vi "Controller Test Bench (15).vi"() -> ()   [LabVIEW 2022 SP3]
uses:
  WhiteNoise.ctl
  <vilib>/sound2/lvsound2.llb/Sound Data Format.ctl
  <vilib>/Utility/error.llb/DialogType.ctl
  <vilib>/sound2/lvsound2.llb/Sampling Mode.ctl
  <vilib>/Platform/TimedLoop/XDataNode/timing_clust.ctl
  <vilib>/Platform/TimedLoop/XDataNode/nitl_modes.ctl
  <vilib>/Platform/TimedLoop/XDataNode/wakeup.ctl
  <vilib>/sound2/lvsound2.llb/Sound File Refnum.ctl
  <vilib>/Analysis/4window.llb/windowTd.ctl
  <vilib>/DAQmx/write.llb/DAQmx Write (Analog 1D Wfm NChan NSamp).vi
  <vilib>/DAQmx/read.llb/DAQmx Read (Analog 1D Wfm NChan NSamp).vi
  <vilib>/DAQmx/create/channels.llb/DAQmx Create Channel (AI-Acceleration-Accelerometer).vi
  <vilib>/DAQmx/configure/timing.llb/DAQmx Timing (Sample Clock).vi
  <vilib>/Platform/TimedLoop/scheduler/LVUserAPI/_suppVIs/Create_1kHz_TSource.vi
  <vilib>/DAQmx/create/channels.llb/DAQmx Create Channel (AO-Voltage-Basic).vi
  <vilib>/sound2/lvsound2.llb/Sound File Info (path).vi
  <vilib>/sound2/lvsound2.llb/Sound File Read Open.vi
  <vilib>/sound2/lvsound2.llb/Sound Output Set Volume (Single).vi
  <vilib>/sound2/lvsound2.llb/Sound File Read (DBL).vi
  <vilib>/sound2/lvsound2.llb/Sound Output Write (DBL).vi
  <vilib>/DAQmx/miscellaneous.llb/DAQmx Fill In Error Info.vi
  <vilib>/DAQmx/configure/task.llb/DAQmx Configure Logging (TDMS).vi
  <vilib>/measure/maspectr.llb/FFT Spectrum (Mag-Phase) for N Chan.vi
  <vilib>/platform/TimedLoop/XDataNode/XDataNode.xnode
  <vilib>/measure/NI_MAPro.lvlib
  <resource>/objmgr/daqmx.rc
  <vilib>/Analysis/NI_AALPro.lvlib
  <vilib>/measure/NI_MABase.lvlib
  <vilib>/addons/control/pid/NI_PID_pid.lvlib
  <vilib>/Platform/TimedLoop/XDataNode/XDNodeRunTimeDep.lvlib
  <vilib>/addons/control/pid/pid.llb/PID (DBL Array).vi
panel:
  in  "Time Out (s)":dbl=1000.0
  out "Elapsed Time":i32 caption="Elapsed Time (s)" format="%.2f"
  in  "Time Out (s)":dbl=1000.0
  out "Active Controller Output":dbl[](graph)
  out "Elapsed Time":i32 caption="Elapsed Time (s)" format="%.2f"
  in  "Acquisition\nPeriod(ms)":dbl=41.2
  out "Accel.1":waveform(dbl)[](graph)
  out "Excitation Output":waveform(dbl)[](graph)
  in  "Output Noise":bool=TRUE
  in  "?":T1(tab)=enum."Harmonic"
  in  "Cluster 3":T2={"Path txt/csv File"=path "C:/Users/LAV-UFSC-2023/Documents/LAV-TCC/Dados-Experimentos/acc_time/Previous Data/handlebar_acc1_run2.txt", "Delimiter"=".", "Separator"="\\t", "Offset (lines)"=21.0}
  in  "Gain":i32
  in  "Stop 3":bool
  in  "Gain":i32
  in  "Cluster 4":T4={"Seed"=0.0, "Iterator"=1.0, "Path Sound File"=path "C:/Users/LAV-UFSC-2023/Documents/LAV-TCC/Dados-Experimentos/Dados Empíricos/Uni-cheio.wav", "number of samples/ch (-1: all)"=-1}
  in  "Stop 2":bool
  in  "Cluster":T5={"Seed"=0.0, "Standard Deviation"=0.2, "Reset"=FALSE, "Iterator"=1.0, "Seed"=-1, "Stop 4"=FALSE, "Lower Cut-Off 2"=5.0, "Upper Cut-Off 2"=350.0} {"Upper Cut-Off 2" min=5.0 max=350.0 step=10.0; "Lower Cut-Off 2" min=5.0 max=350.0 step=10.0; "Standard Deviation" min=0.001 max=1.5 step=0.05 format="%0.2p"}
  in  "Cluster 2":T6={"Iterator"=1.0, "Waveform Type"=0, "Frequency"=10.0, "Amplitude"=0.25, "Stop 4"=FALSE} {"Frequency" min=5.0 max=350.0 step=10.0 format="%0.2p"; "Waveform Type" items=["Sine Wave", "Triangle Wave", "Square Wave", "Sawtooth Wave"]; "Amplitude" min=0.001 max=0.3 step=0.05 format="%0.2p"}
  in  "Active Control":bool
  in  "Tab Control":T7(tab)
  out "dt out (s)":dbl format="%.3f"
  in  "setpoint":dbl[](array[numeric])=[0.0] format="%.2f"
  in  "PID gains":T8(array[cluster])=[{"proportional gain (Kc)"=1.0, "integral time (Ti, min)"=0.01, "derivative time (Td, min)"=0.0}] {"derivative time (Td, min)" format="%.3e"; "integral time (Ti, min)" format="%.3e"; "proportional gain (Kc)" step=0.0025 format="%.3e"}
  in  "dt (s)":dbl=-1.0 format="%.3f"
  in  "output range":cluster{"output high":dbl, "output low":dbl}[](array[cluster])=[{"output high"=100.0, "output low"=-100.0}] {"output low" format="%.2f"; "output high" format="%.2f"}
  in  "Upper Cut-Off":dbl=400.0
  in  "Lower Cut-Off":dbl=100.0
  in  "Setpoint":dbl
  in  "Gain":dbl min=0.0 step=0.01
  out "Output Signal":dynamicdata(graph)
  in  "Upper Cut-Off":dbl=400.0
  in  "Lower Cut-Off":dbl=100.0
  out "Accel.2":waveform(dbl)[](graph)
  in  "Log Raw Data":bool
  out "Mag 2":cluster{"f0":dbl, "df":dbl, "magnitude":dbl[]}[](graph)
  in  "Show FFT":bool=TRUE
  in  "Log FFT":bool
  in  "Start Reading":bool=TRUE
  in  "Stop":bool
  # "Active Controller"
  # "Main\nSwitch"
  # "Output Noise"
  # "RAW - Accel. 1"
  # "Data Acquisition"
  # "FFT - Amplitude (dB)"
  # "RAW - Accel. 2"
  # "Runtime"
  # "Pre-Set"
  # "Runtime"
  # "Pre-Set"
  # "Runtime"
  # "Filter"
  # "Runtime"
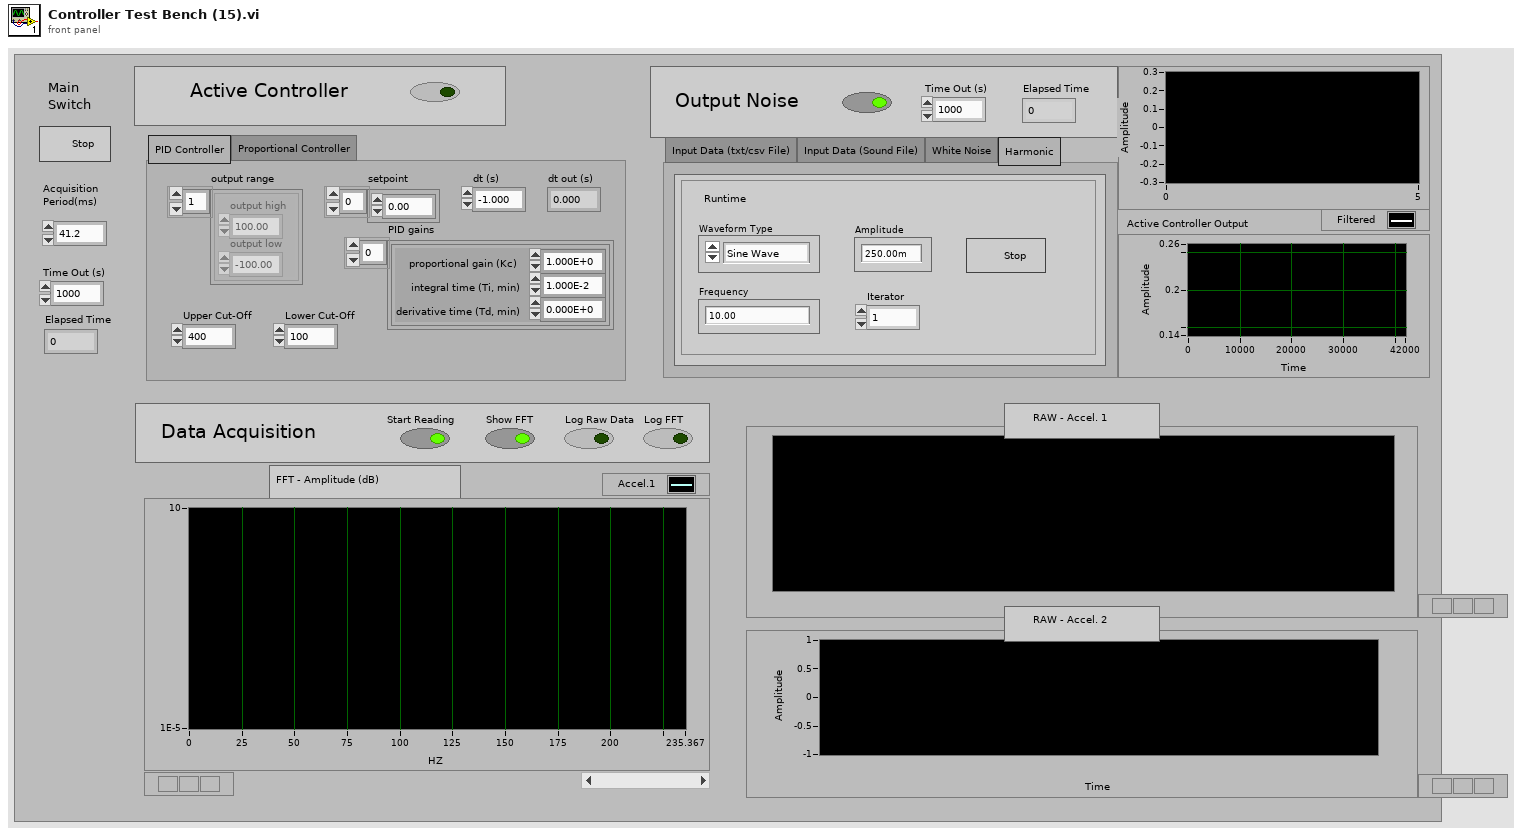
[diagram p1: front panel]
types:
  T1 = enum32{"Input Data (txt/csv File)", "Input Data (Sound File)", "White Noise", "Harmonic"}
  T2 = cluster{"Path txt/csv File":path, "Delimiter":string, "Separator":string, "Offset (lines)":dbl}
  T3 = typedef "WhiteNoise.ctl" = dbl
  T4 = cluster{"Seed":T3, "Iterator":dbl, "Path Sound File":path, "number of samples/ch (-1: all)":i32}
  T5 = cluster{"Seed":T3, "Standard Deviation":dbl, "Reset":bool, "Iterator":dbl, "Seed":i8, "Stop 4":bool, "Lower Cut-Off 2":dbl, "Upper Cut-Off 2":dbl}
  T6 = cluster{"Iterator":dbl, "Waveform Type":u16, "Frequency":dbl, "Amplitude":dbl, "Stop 4":bool}
  T7 = enum32{"PID Controller", "Proportional Controller"}
  T8 = cluster{"proportional gain (Kc)":dbl, "integral time (Ti, min)":dbl, "derivative time (Td, min)":dbl}[]
  T9 = typedef "Sampling Mode.ctl" = i32
  T10 = typedef "DialogType.ctl" = u16
  T11 = typedef "Sound Data Format.ctl" = cluster{"sample rate (S/s)":dbl, "number of channels":i32, "bits per sample":i32}
  T12 = typedef "Sound Output Task ID.ctl" = u32
  T13 = typedef "XDNodeRunTimeDep.lvlib/timing_clust.ctl" = cluster{"Expected End [f-1]":u64, "Actual End [f-1]":u64, "Finished Late? [f-1]":bool, "Expected End [i-1]":u64, "Actual End [i-1]":u64, "Finished Late? [i-1]":bool, "Expected Start [i]":u64, "Actual Start [i]":u64, "Expected Start [f]":u64, "Actual Start [f]":u64, "Source Name":string, "Structure Name":string, "Period":i64, "Deadline":i64, "Offset":i64, "Start":i64, "Priority":i32, "Timeout":i32, "Mode":T14, "Wakeup Reason":T15, "Error":errorcluster, "Source Type":string, "Secondary Source Type":string, "Global End Time":u64, "Global Start Time":u64, "Frame Duration":u64, "Iteration Duration":u64, "Assigned CPU":i32, "I/O Scan Engine Mode":u32}
  T14 = typedef "XDNodeRunTimeDep.lvlib/nitl_modes.ctl" = enum32{"No Change", "Process missed periods, maintain original phase", "Discard missed periods, maintain original phase", "Process missed periods, ignore original phase", "Discard missed periods, ignore original phase"}
  T15 = typedef "XDNodeRunTimeDep.lvlib/wakeup.ctl" = enum32{"Normal", "Aborted", "Asynchronous wakeup", "Timing source error", "Timed loop error", "Timeout"}
  T16 = typedef "Sound File Refnum.ctl" = refnum<file>
  T17 = typedef "NI_AALPro.lvlib/windowTd.ctl" = u32
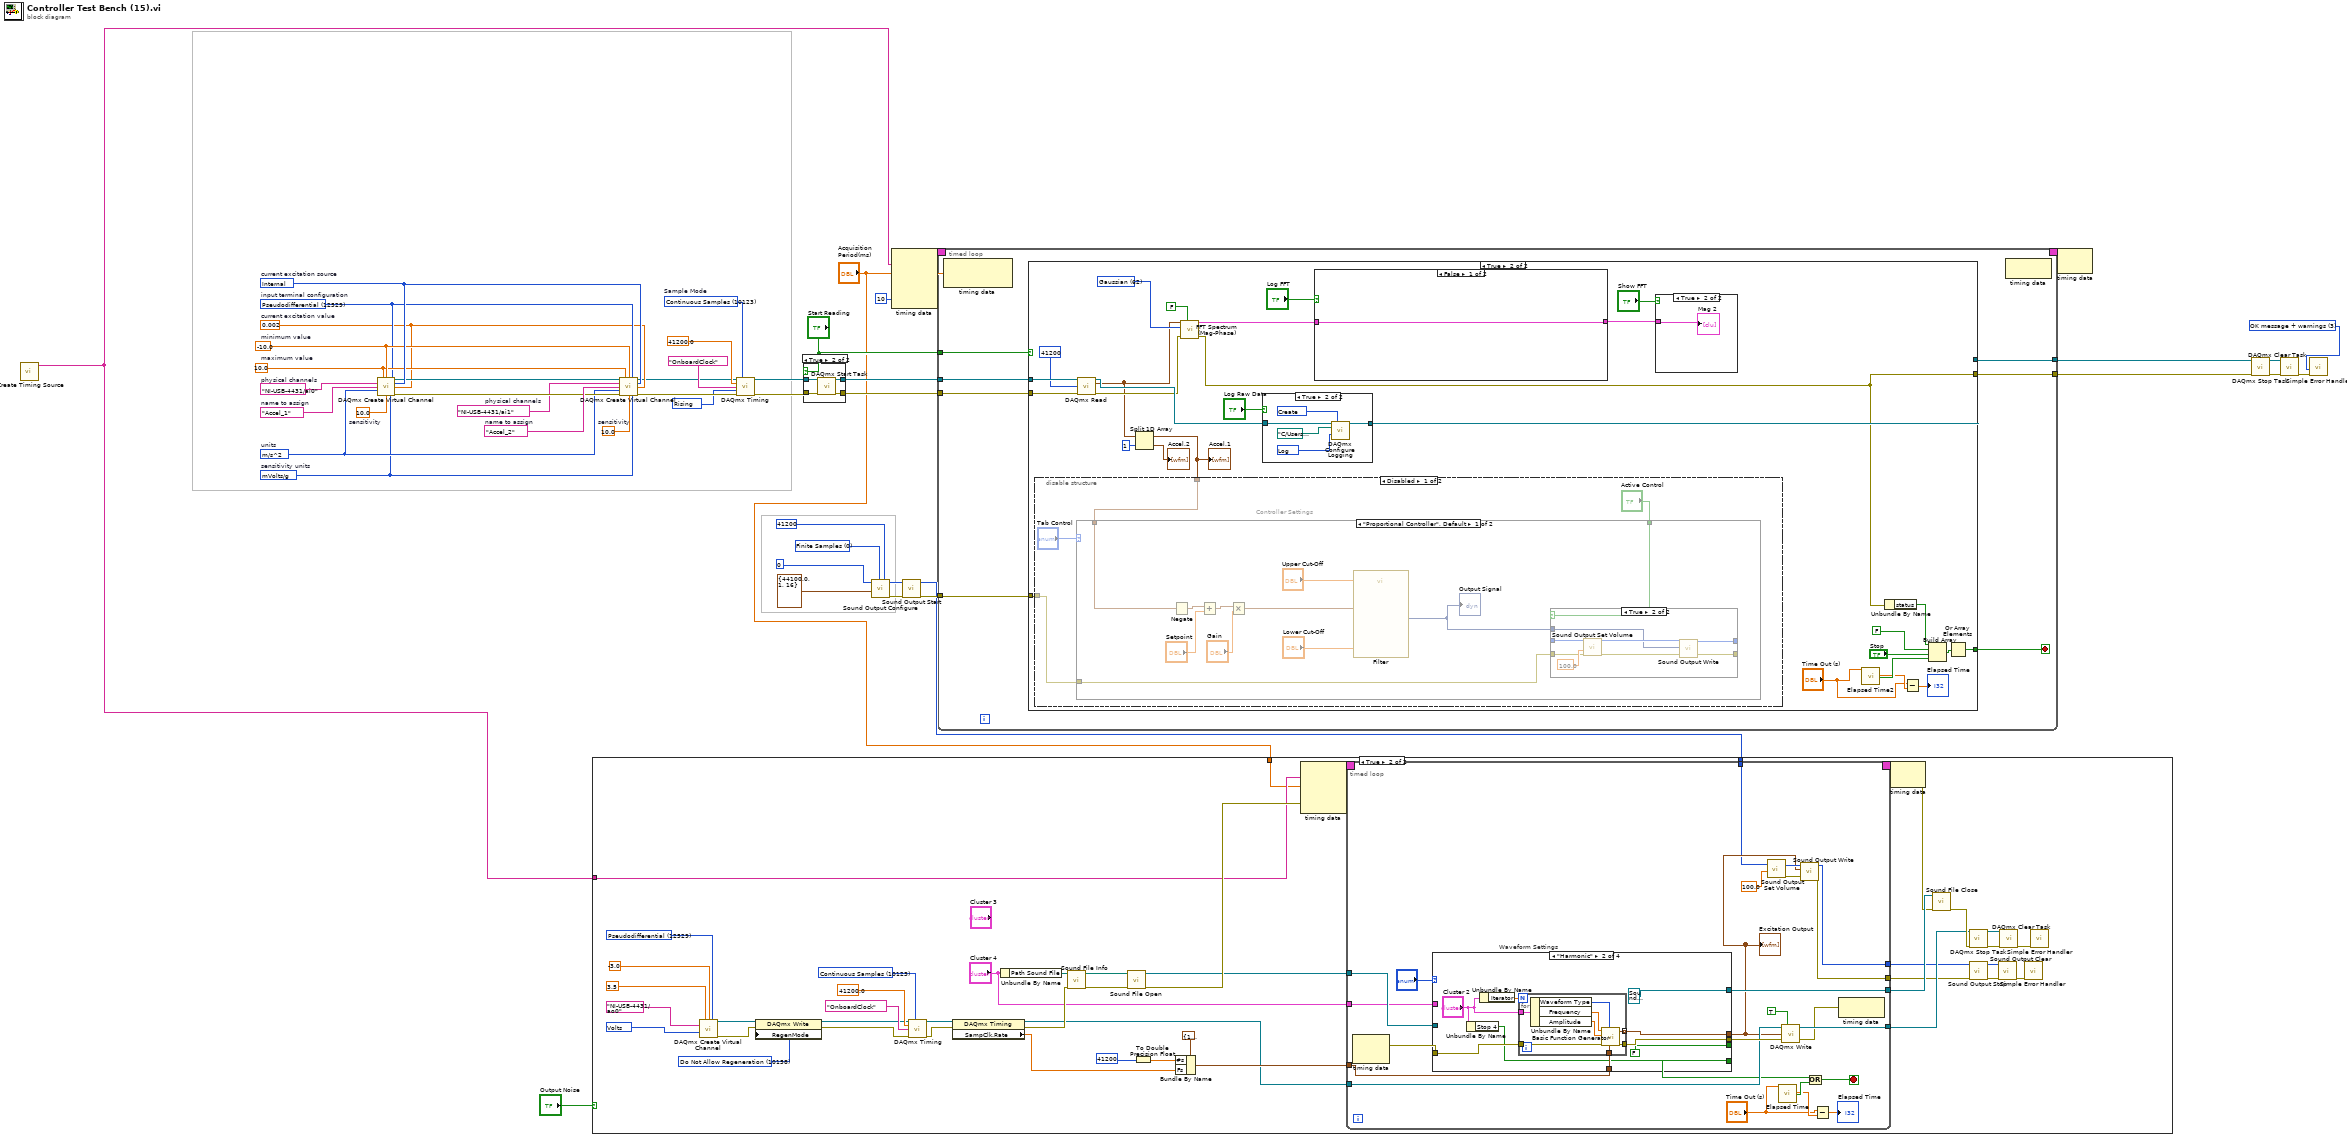
[diagram p0: block diagram]
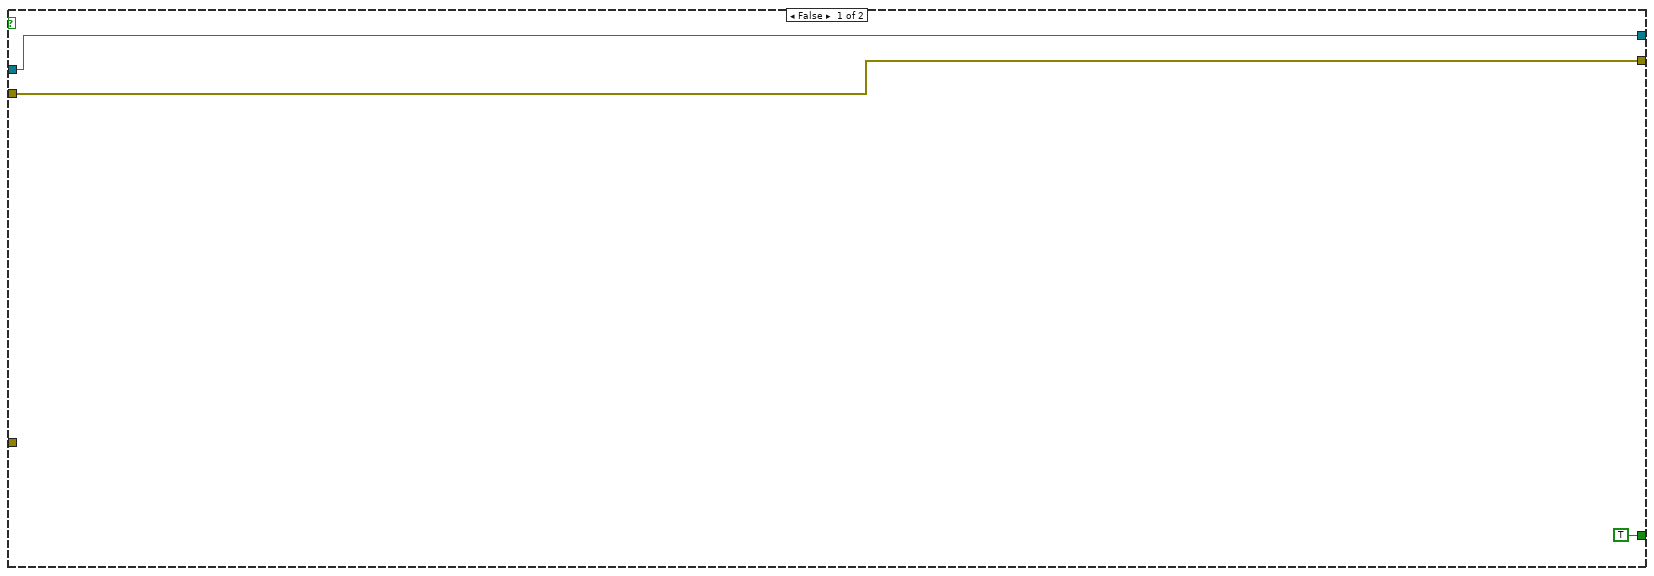
[diagram p2: hidden frame]
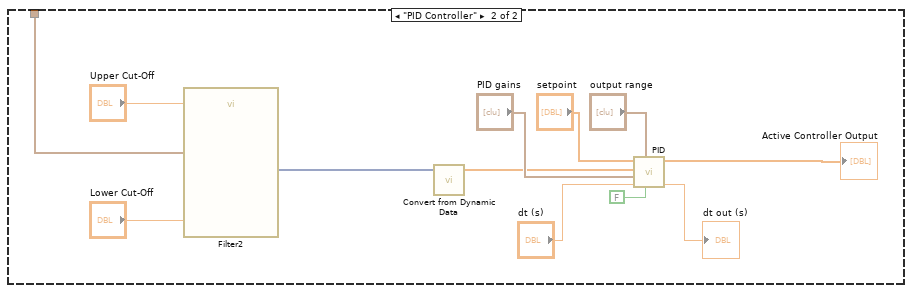
[diagram p4: hidden frame]
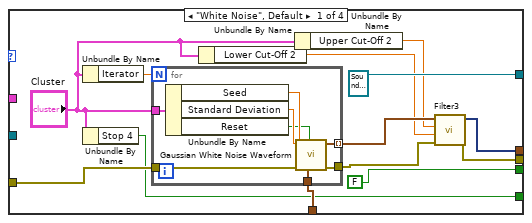
[diagram p10: hidden frame]
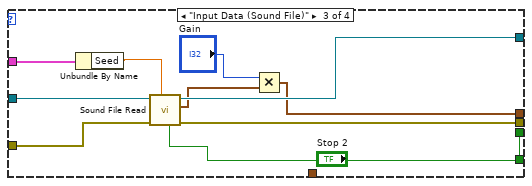
[diagram p11: hidden frame]
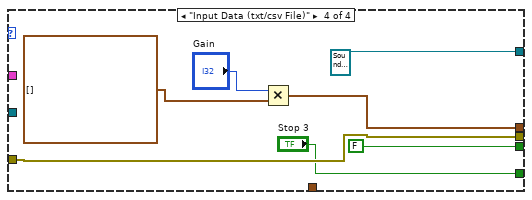
[diagram p12: hidden frame]
diagram:
  w4 = 10280 items=["Rising"=10280, "Falling"=10171] ("active edge")
  w6 = 12509 items=["mVolts/g"=12509, "Volts/g"=12510]  # sensitivity units
  w35 = 10.0  # sensitivity
  w5 = 0.002  # current excitation value
  w29 = 10200 items=["Internal"=10200, "External"=10167, "None"=10230]  # current excitation source
  w21 = tag "NI-USB-4431/ai0"  # physical channels
  w34 = 10123 items=["Finite Samples"=10178, "Continuous Samples"=10123, "Hardware Timed Single Point"=12522]  # Sample Mode
  w24 = 12529 items=["default"=-1, "RSE"=10083, "NRSE"=10078, "Differential"=10106, "Pseudodifferential"=12529]  # input terminal configuration
  w27 = -10.0  # minimum value
  w26 = 10.0  # maximum value
  w36 = "Accel_1"  # name to assign
  w25 = 12470 items=["g"=10186, "m/s^2"=12470, "in/s^2"=12471, "From Custom Scale"=10065]  # units
  w37 = 10.0  # sensitivity
  w22 = tag "NI-USB-4431/ai1"  # physical channels
  w31 = "Accel_2"  # name to assign
  w38 = T9 0 items=["Finite Samples", "Continuous Samples"] ("sample mode")
  w39 = T10 3 items=["no dialog", "OK message", "continue or stop message", "OK message + warnings", "continue/stop + warnings"] ("type of dialog (OK msg:1)")
  n1 = call-poly <vilib>:"Create Timing Source.vi"() -> ("name (out)"=w13:string)  [unwired: 10 in, 1 out]
  n2 = call-poly <vilib>:"DAQmx Create Virtual Channel.vi"("maximum value"=w26, "minimum value"=w27, "input terminal configuration"=w24, "physical channels"=w21, "current excitation source"=w29, "name to assign"=w36, "current excitation value"=w5, "units"=w25, "sensitivity"=w35, "sensitivity units"=w6) -> ("task out"=w23:refnum<k21>, "error out"=w30:errorcluster)  [unwired: 4 in]
  n3 = call-poly <vilib>:"DAQmx Create Virtual Channel.vi"("task in"=w23, "maximum value"=w26, "minimum value"=w27, "input terminal configuration"=w24, "physical channels"=w22, "current excitation source"=w29, "name to assign"=w31, "current excitation value"=w5, "units"=w25, "error in"=w30, "sensitivity"=w37, "sensitivity units"=w6) -> ("task out"=w2:refnum<k21>, "error out"=w28:errorcluster)  [unwired: 2 in]
  n4 = call-poly <vilib>:"DAQmx Timing.vi"("task/channels in"=w2, "sample mode"=w34, "rate"=41200.0 ("Sample Rate"), "source"=tag "OnboardClock" ("Sample Clock Source"), "active edge"=w4, "error in"=w28) -> ("task out"=w19:refnum<k21>, "error out"=w20:errorcluster)  [unwired: 8 in]
  n5 = case shown="True" "Start Reading" {
    tunnel: w20 -> [w47 w52]
    tunnel: w19 -> [w48 w51]
    tunnel: [w48 w50] -> w10
    tunnel: [w47 w49] -> w11
    frame False {
    }
    frame True {
      n6 = call <vilib>:"DAQmx Start Task.vi"("task/channels in"=w51, "error in"=w52) -> ("task out"=w50:refnum<k21>, "error out"=w49:errorcluster)  [unwired: 12 in]
    }
  }
  n7 = call <vilib>:"Sound Output Configure.vi"("number of samples/ch"=41200 ("Number of Samples/ch"), "sample mode"=w38, "sound format"=T11 {"sample rate (S/s)"=44100.0, "number of channels"=1, "bits per sample"=16} ("Sound Format"), "device ID"=u32 0 ("Device ID")) -> ("error out"=w18:errorcluster, "task ID"=w17:T12)  [unwired: 6 in]
  n8 = node-c288(w13, "Acquisition\nPeriod(ms)", i64 10 ("Offset")) -> (w15:T13)  [unwired: 2 in]
  n9 = call <vilib>:"Sound Output Start.vi"("error in (no error)"=w18, "task ID"=w17) -> ("error out"=w12:errorcluster, "task ID out"=w1:T12)  [unwired: 8 in]
  n10 = case shown="True" "Output Noise" {
    tunnel: w13 -> [_ w69]
    tunnel: "Acquisition\nPeriod(ms)" -> [_ w59]
    tunnel: w1 -> [_ w53]
    frame False {
    }
    frame True {
      w85 = 10123 items=["Finite Samples"=10178, "Continuous Samples"=10123, "Hardware Timed Single Point"=12522] ("sample mode")
      w89 = 10158 items=["Allow Regeneration"=10097, "Do Not Allow Regeneration"=10158] ("RegenMode")
      w95 = 12529 items=["Default"=-1, "RSE"=10083, "Differential"=10106, "Pseudodifferential"=12529] ("output terminal configuration")
      w93 = 10348 items=["Volts"=10348, "From Custom Scale"=10065] ("units")
      n11 = call-poly <vilib>:"DAQmx Create Virtual Channel.vi"("maximum value"=3.5, "minimum value"=-3.0, "output terminal configuration"=w95, "physical channels"=tag "NI-USB-4431/ao0", "units"=w93) -> ("task out"=w88:refnum<k21>, "error out"=w90:errorcluster)  [unwired: 9 in]
      n12 = property class="DAQmx Write"(reference=w88, error in=w90, "RegenMode"=w89) -> (reference out=w86:refnum<k21>, error out=w87:errorcluster)
      n13 = call-poly <vilib>:"DAQmx Timing.vi"("task/channels in"=w86, "sample mode"=w85, "rate"=41200.0 ("Sample Rate"), "source"=tag "OnboardClock" ("Sample Clock Source"), "error in"=w87) -> ("task out"=w81:refnum<k21>, "error out"=w80:errorcluster)  [unwired: 9 in]
      n14 = property class="DAQmx Timing"(reference=w81, error in=w80) -> (reference out=w64:refnum<k21>, error out=w74:errorcluster, "SampClk.Rate"=w82:dbl)
      n15 = Unbundle By Name("Cluster 4") -> ("Path Sound File"=w62:path)
      n16 = call-poly <vilib>:"Sound File Info.vi"("error in (no error)"=w74, "path"=w62) -> ("error out"=w76:errorcluster, "path out"=w75:path)  [unwired: 6 in, 2 out]
      n17 = call-poly <vilib>:"Sound File Open.vi"("error in (no error)"=w76, "path"=w75) -> ("error out"=w70:errorcluster, "sound file refnum"=w68:T16)  [unwired: 8 in]
      n18 = To Double Precision Float(number=41200) -> (double precision float=w83:dbl)
      n19 = Bundle By Name(cluster=cluster{"Fs":dbl, "#s":dbl} {"Fs"=1000.0, "#s"=1000.0} ("sampling info"), "#s"=w83, "Fs"=w82) -> (w65:cluster{"Fs":dbl, "#s":dbl})
      n20 = node-c288(w69, w59, w70) -> (w72:T13)  [unwired: 1 in]
      n21 = timed-loop {
        timing: w72 -> [_]
        timing-out: [_] -> w71
        tunnel: w68 -> [w117]
        tunnel: [w116] -> w67
        tunnel: [w115] -> w66
        tunnel: w65 -> [w114]
        tunnel: w64 -> [w113]
        tunnel: "Cluster 4" -> [w112]
        tunnel: [w100] -> w55
        tunnel: [w99] -> w54
        tunnel: w53 -> [w98]
        stop <- w111 stop-if-true
        # "Waveform Settings"
        n22 = node-c288() -> (w118:errorcluster)  [unwired: 1 in, 1 out]
        n23 = case shown="\"Harmonic\"" "?" {
          tunnel: w114 -> [w134 w149 _ _]
          tunnel: w118 -> [w132 w151 w170 w175]
          tunnel: [w125 w148 w169 w175] -> w120
          tunnel: [w127 w150 w165 w171] -> w101
          tunnel: w117 -> [_ _ w168 _]
          tunnel: [FALSE FALSE w167 FALSE ("end of file?")] -> _
          tunnel: [T16 refnum ("sound file refnum out") T16 refnum ("sound file refnum out") w166 T16 refnum ("sound file refnum out")] -> w116
          tunnel: w112 -> [_ _ w162 _]
          tunnel: [w129 w143 "Stop 2" "Stop 3"] -> w110
          frame "White Noise", Default {
            n24 = Unbundle By Name("Cluster") -> ("Iterator"=w133:dbl)
            n25 = Unbundle By Name("Cluster") -> ("Stop 4"=w129:bool)
            n26 = for {
              N: w133 -> [_]
              tunnel: w132 -> [w142]
              tunnel: w134 -> [w141]
              tunnel: [w140] -> w126
              tunnel: "Cluster" -> [w139]
              tunnel: [w138] -> w128 mode=indexing
              n27 = Unbundle By Name(w139) -> ("Seed"=w137:T3, "Standard Deviation"=w136:dbl, "Reset"=w135:bool)
              n28 = call <vilib>:"Gaussian White Noise Waveform.vi"("sampling info"=w141, "reset signal"=w135, "error in (no error)"=w142, "seed"=w137, "standard deviation"=w136) -> ("error out"=w140:errorcluster, "signal out"=w138:waveform(dbl))  [unwired: 5 in]
            }
            n29 = Unbundle By Name("Cluster") -> ("Lower Cut-Off 2"=w123:dbl)
            n30 = Unbundle By Name("Cluster") -> ("Upper Cut-Off 2"=w122:dbl)
            n31 = call "Filter3"("error in (no error)"=w126, "Lower Cut-Off"=w123, "Upper Cut-Off"=w122, "Signal"=w128) -> ("error out"=w125:errorcluster, "Filtered Signal"=w127:dynamicdata)  [unwired: 6 in]
          }
          frame "Harmonic" {
            n32 = Unbundle By Name("Cluster 2") -> ("Stop 4"=w143:bool)
            n33 = Unbundle By Name("Cluster 2") -> ("Iterator"=w147:dbl)
            n34 = for {
              N: w147 -> [_]
              tunnel: w151 -> [w159]
              tunnel: w149 -> [w158]
              tunnel: [w157] -> w148
              tunnel: "Cluster 2" -> [w156]
              tunnel: [w152] -> w150 mode=indexing
              n35 = Unbundle By Name(w156) -> ("Waveform Type"=w155:u16, "Frequency"=w154:dbl, "Amplitude"=w153:dbl)
              n36 = call <vilib>:"Basic Function Generator.vi"("sampling info"=w158, "signal type"=w155, "error in (no error)"=w159, "amplitude"=w153, "frequency"=w154) -> ("error out"=w157:errorcluster, "signal out"=w152:waveform(dbl))  [unwired: 4 in, 1 out]
            }
          }
          frame "Input Data (Sound File)" {
            n37 = Unbundle By Name(w162) -> ("Seed"=w163:T3)
            n38 = call-poly <vilib>:"Sound File Read.vi"("number of samples/ch (-1: all)"=w163, "error in (no error)"=w170, "sound file refnum"=w168) -> ("error out"=w169:errorcluster, "data"=w164:waveform(dbl)[], "sound file refnum out"=w166:T16, "end of file?"=w167:bool)  [unwired: 4 in, 1 out]
            n39 = Multiply(x="Gain", y=w164) -> (x*y=w165:waveform(dbl)[])
          }
          frame "Input Data (txt/csv File)" {
            n40 = Multiply(x="Gain", y=waveform(dbl)[] []) -> (x*y=w171:waveform(dbl)[])
          }
        }
        "Excitation Output" <- w101
        n41 = call-poly <vilib>:"Sound Output Set Volume.vi"("volume"=100.0, "task ID"=w98) -> ("error out"=w102:errorcluster, "task ID out"=w103:T12)  [unwired: 8 in]
        n42 = call "Elapsed Time"("Time Target (s)"="Time Out (s)") -> ("Elapsed Time (s)"=w106:dbl, "Time has Elapsed"=w107:bool)  [unwired: 11 in, 6 out]
        n43 = call-poly <vilib>:"DAQmx Write.vi"("task/channels in"=w113, "auto start"=TRUE, "data"=w101, "error in"=w120) -> ("task out"=w115:refnum<k21>, "error out"=w109:errorcluster)  [unwired: 9 in, 1 out]
        n44 = call-poly <vilib>:"Sound Output Write.vi"("error in (no error)"=w102, "data"=w101, "task ID"=w103) -> ("error out"=w99:errorcluster, "task ID out"=w100:T12)  [unwired: 7 in]
        n45 = Or(x=w110, y=w107) -> (x .or. y?=w111:bool)
        n46 = Subtract(x="Time Out (s)", y=w106) -> (x-y=→"Elapsed Time":dbl)
        n47 = node-c288(w109) -> ()  [unwired: 1 out]
      }
      n48 = node-c288(w71) -> (w60:errorcluster)
      n49 = call <vilib>:"Sound File Close.vi"("error in (no error)"=w60, "sound file refnum"=w67) -> ("error out"=w73:errorcluster)  [unwired: 9 in]
      n50 = call <vilib>:"DAQmx Stop Task.vi"("task/channels in"=w66, "error in"=w73) -> ("task out"=w79:refnum<k21>, "error out"=w78:errorcluster)  [unwired: 12 in]
      n51 = call <vilib>:"Sound Output Stop.vi"("error in (no error)"=w54, "task ID"=w55) -> ("error out"=w56:errorcluster, "task ID out"=w57:T12)  [unwired: 8 in]
      n52 = call <vilib>:"Sound Output Clear.vi"("error in (no error)"=w56, "task ID"=w57) -> ("error out"=w58:errorcluster)  [unwired: 9 in]
      n53 = call <vilib>:"DAQmx Clear Task.vi"("task in"=w79, "error in"=w78) -> ("error out"=w77:errorcluster)  [unwired: 13 in]
      n54 = call <vilib>:"Simple Error Handler.vi"("error in (no error)"=w58) -> ()  [unwired: 4 in, 5 out]
      n55 = call <vilib>:"Simple Error Handler.vi"("error in (no error)"=w77) -> ()  [unwired: 4 in, 5 out]
    }
  }
  n56 = timed-loop {
    timing: w15 -> [_]
    timing-out: [_] -> w14
    tunnel: "Start Reading" -> [w196]
    tunnel: w12 -> [w195]
    tunnel: w11 -> [w194]
    tunnel: w10 -> [w193]
    tunnel: [w192] -> w9
    tunnel: [w191] -> w8
    stop <- w190 stop-if-true
    n57 = node-c288() -> ()  [unwired: 1 in, 2 out]
    n58 = case shown="True" w196 {
      tunnel: w193 -> [w199 w227]
      tunnel: w194 -> [w198 w226]
      tunnel: [w199 w223] -> w191
      tunnel: [w198 w214] -> w192
      tunnel: w195 -> [_ w208]
      tunnel: [TRUE w205] -> w190
      frame False {
      }
      frame True {
        w213 = T17 62 items=["Rectangle"=0, "Hanning"=1, "Hamming"=2, "Blackman-Harris"=3, "Exact Blackman"=4, "Blackman"=5, "Flat Top"=6, "4 Term B-Harris "=7, "7 Term B-Harris"=8, "Low Sidelobe"=9, "Blackman Nuttall"=11, "Triangle"=30, "Bartlett-Hanning"=31, "Bohman"=32, "Parzen"=33, "Welch"=34, "Kaiser"=60, "Dolph-Chebyshev"=61, "Gaussian"=62] ("window")
        n59 = call-poly <vilib>:"DAQmx Read.vi"("task/channels in"=w227, "number of samples per channel"=41200, "error in"=w226) -> ("task out"=w224:refnum<k21>, "data"=w207:waveform(dbl)[], "error out"=w215:errorcluster)  [unwired: 10 in]
        n60 = Split 1D Array(array=w207, index=1) -> (first subarray=w206:waveform(dbl)[], second subarray=→"Accel.2":waveform(dbl)[])
        "Accel.1" <- w206
        n61 = disable-structure shown="Disabled" {
          disable-tunnel: w208 -> [w230 _]
          disable-tunnel: w206 -> [w228 _]
          frame Disabled {
            # "Controller Settings"
            n62 = case shown="\"Proportional Controller\", Default" "Tab Control" {
              tunnel: w228 -> [w238 w253]
              tunnel: w230 -> [w237 _]
              tunnel: "Active Control" -> [w236 _]
              frame "Proportional Controller", Default {
                n63 = Negate(x=w238) -> (-x=w241:waveform(dbl)[])
                n64 = Add(x=w241, y="Setpoint") -> (x+y=w240:waveform(dbl)[])
                n65 = Multiply(x=w240, y="Gain") -> (x*y=w235:waveform(dbl)[])
                n66 = call "Filter"("Lower Cut-Off"="Lower Cut-Off", "Upper Cut-Off"="Upper Cut-Off", "Signal"=w235) -> ("Filtered Signal"=w234:dynamicdata)  [unwired: 7 in, 1 out]
                "Output Signal" <- w234
                n67 = case shown="True" w236 {
                  tunnel: w237 -> [w244 w251]
                  tunnel: [w244 w248] -> _
                  tunnel: _ -> [w243 w245]
                  tunnel: [w243 w247] -> _
                  tunnel: w234 -> [_ w246]
                  frame False {
                  }
                  frame True {
                    n68 = call-poly <vilib>:"Sound Output Set Volume.vi"("error in (no error)"=w251, "volume"=100.0, "task ID"=w245) -> ("error out"=w249:errorcluster, "task ID out"=w250:T12)  [unwired: 7 in]
                    n69 = call-poly <vilib>:"Sound Output Write.vi"("error in (no error)"=w249, "data"=w246, "task ID"=w250) -> ("error out"=w248:errorcluster, "task ID out"=w247:T12)  [unwired: 7 in]
                  }
                }
              }
              frame "PID Controller" {
                n70 = call "Filter2"("Lower Cut-Off"="Lower Cut-Off", "Upper Cut-Off"="Upper Cut-Off", "Signal"=w253) -> ("Filtered Signal"=w255:dynamicdata)  [unwired: 7 in, 1 out]
                n71 = call "Convert from Dynamic Data"("Dynamic Data Type"=w255) -> ("Array"=w254:dbl[])  [unwired: 3 in]
                n72 = call-poly <vilib>:"PID.vi"("reinitialize? (F)"=FALSE, "output range"="output range", "dt (s)"="dt (s)", "PID gains"="PID gains", "process variable"=w254, "setpoint"="setpoint") -> ("dt out (s)"=→"dt out (s)":dbl, "output"=→"Active Controller Output":dbl[])  [unwired: 4 in]
              }
            }
          }
          frame Enabled {
          }
        }
        n73 = call-poly <vilib>:"FFT Spectrum (Mag-Phase).vi"("restart averaging (F)"=FALSE, "error in (no error)"=w215, "window"=w213, "time signals"=w207) -> ("error out"=w214:errorcluster, "magnitudes"=w218:cluster{"f0":dbl, "df":dbl, "magnitude":dbl[]}[])  [unwired: 3 in, 3 out]
        n74 = case shown="True" "Log Raw Data" {
          tunnel: w224 -> [w268 w270]
          tunnel: [w268 w269] -> w223
          frame False {
          }
          frame True {
            w271 = 15848 items=["Open"=10437, "Open or Create"=15846, "Create or Replace"=15847, "Create"=15848] ("operation")
            w272 = 15844 items=["Off"=10231, "Log"=15844, "Log and Read"=15842] ("logging mode")
            n75 = call-poly <vilib>:"DAQmx Configure Logging.vi"("task/channels in"=w270, "operation"=w271, "file path"=path "C:/Users/LAV-UFSC/Documents/LAV - TCC", "logging mode"=w272) -> ("task out"=w269:refnum<k21>)  [unwired: 10 in, 1 out]
          }
        }
        n76 = case shown="False" "Log FFT" {
          tunnel: w218 -> [w265 w266]
          tunnel: [w265 w266] -> w217
          frame False {
          }
          frame True {
          }
        }
        n77 = case shown="True" "Show FFT" {
          tunnel: w217 -> [_ w267]
          frame False {
          }
          frame True {
            "Mag 2" <- w267
          }
        }
        n78 = call "Elapsed Time2"("Time Target (s)"="Time Out (s)") -> ("Elapsed Time (s)"=w202:dbl, "Time has Elapsed"=w204:bool)  [unwired: 11 in, 6 out]
        n79 = Unbundle By Name(w214) -> ("status"=w211:bool)
        n80 = Subtract(x="Time Out (s)", y=w202) -> (x-y=→"Elapsed Time":dbl)
        n81 = Build Array(w211, FALSE ("element"), "Stop", w204) -> (w221:bool[])
        n82 = Or Array Elements(Boolean array=w221) -> (logical OR=w205:bool)
      }
    }
    n83 = node-c288() -> ()  [unwired: 1 in, 1 out]
  }
  n84 = node-c288(w14) -> ()  [unwired: 1 out]
  n85 = call <vilib>:"DAQmx Stop Task.vi"("task/channels in"=w8, "error in"=w9) -> ("task out"=w42:refnum<k21>, "error out"=w41:errorcluster)  [unwired: 12 in]
  n86 = call <vilib>:"DAQmx Clear Task.vi"("task in"=w42, "error in"=w41) -> ("error out"=w43:errorcluster)  [unwired: 13 in]
  n87 = call <vilib>:"Simple Error Handler.vi"("type of dialog (OK msg:1)"=w39, "error in (no error)"=w43) -> ()  [unwired: 3 in, 5 out]
